vi "题目二.vi"() -> ()   [LabVIEW 2017]
uses:
  <vilib>/Waveform/WDTFileIO.llb/ Write Waveform to File.vi
  <vilib>/Waveform/WDTFileIO.llb/Read Waveform from File.vi
  <vilib>/measure/NI_MABase.lvlib
panel:
  out "波形图":waveform(dbl)(graph)
  out "first waveform in record":waveform(dbl) caption="记录中第一波形"
  out "名称":string
  out "拆分的路径":path
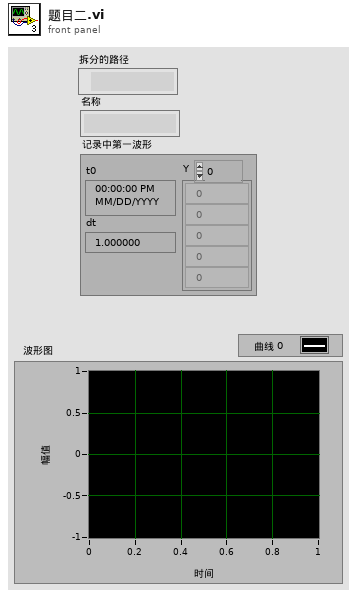
[diagram p1: front panel]
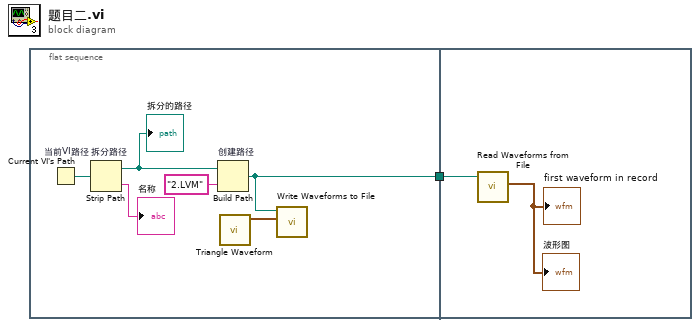
[diagram p0: block diagram]
diagram:
  n1 = flat-sequence {
    tunnel: [w2] -> w1
    tunnel: w1 -> [w9]
    frame #0 {
      n2 = Current VI's Path "当前VI路径"() -> (path=w7:path)
      n3 = Strip Path "拆分路径"(path=w7) -> (stripped path=w5:path, name=→"名称":string)
      "拆分的路径" <- w5
      n4 = Build Path "创建路径"(base path=w5, name or relative path="2.LVM" ("名称或相对路径")) -> (appended path=w2:path)
      n5 = call <vilib>:"Triangle Waveform.vi"() -> ("signal out"=w3:waveform(dbl))  [unwired: 10 in, 1 out]
      n6 = call-poly <vilib>:"Write Waveforms to File.vi"("waveform"=w3, "file path (dialog if empty)"=w2) -> ()  [unwired: 8 in, 2 out]
    }
    frame #1 {
      n7 = call-poly <vilib>:"Read Waveforms from File.vi"("file path (dialog if empty)"=w9) -> ("first waveform in record"=→"first waveform in record" →"波形图":waveform(dbl))  [unwired: 5 in, 3 out]
    }
  }
